vi "Untitled 1.vi"() -> ()   [LabVIEW 2016]
uses:
  BuildItem.ctl
  <vilib>/addons/_JKI.lib/Serialization/JSON/JKI JSON Serialization.lvlib
panel:
  in  "EnableAll":bool
  in  "DisableAll":bool
  in  "Cluster":cluster{"Enable":bool, "BuildItem":T1}={"Enable"=TRUE, "BuildItem"={"Project"=path "", "BuildSpecification"=path "", "Destination"=path ""}}
  in  "OK Button":bool
  in  "Array":cluster{"Enable":bool, "BuildItem":T1}[](array[cluster])
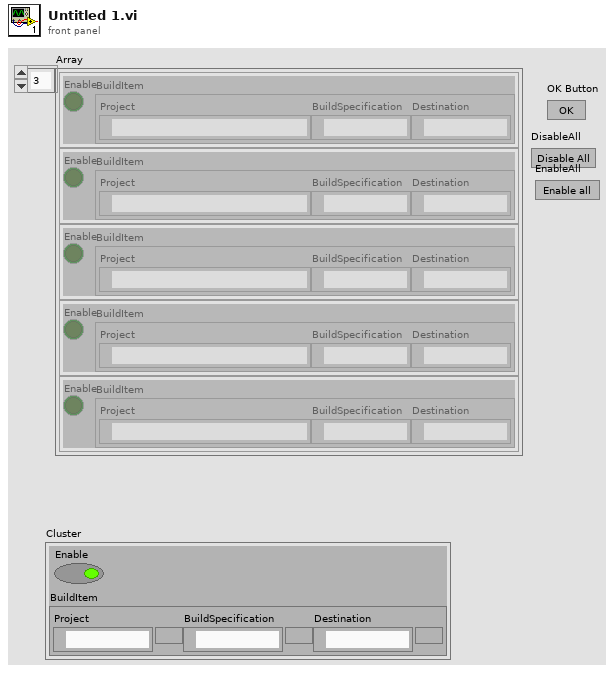
[diagram p1: front panel]
types:
  T1 = typedef "BuildItem.ctl" = cluster{"Project":path, "BuildSpecification":path, "Destination":path}
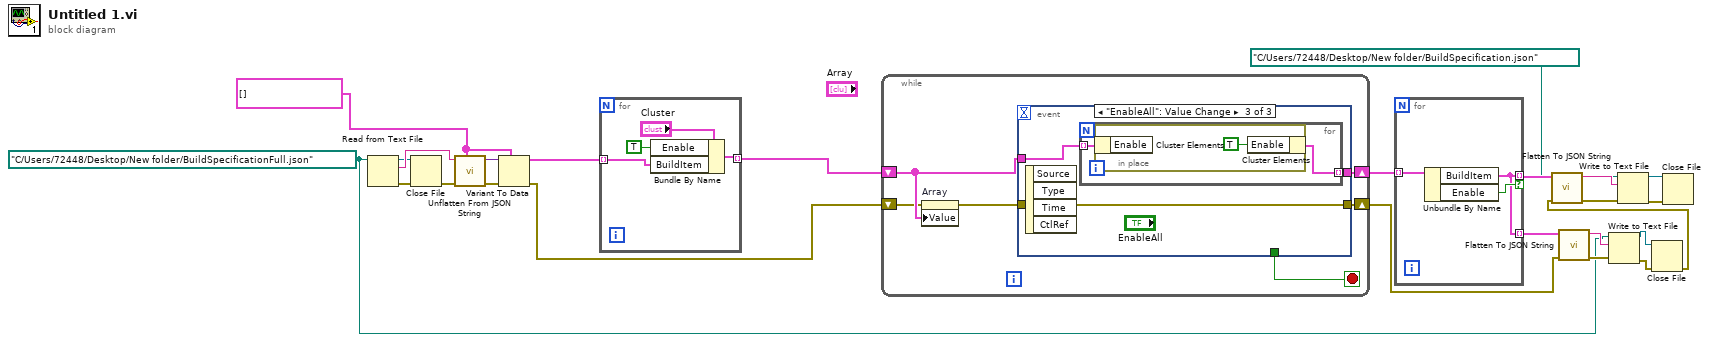
[diagram p0: block diagram]
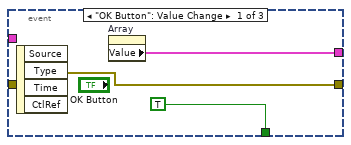
[diagram p2: hidden frame]
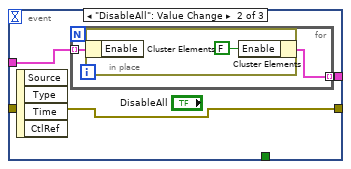
[diagram p3: hidden frame]
diagram:
  w18 = T1[] []
  w4 = path "C:/Users/72448/Desktop/New folder/BuildSpecificationFull.json" ("file (use dialog)")
  n1 = Read from Text File(file (use dialog)=w4) -> (refnum out=w20:refnum<file>, text=w23:string, error out=w21:errorcluster)  [unwired: 3 in, 1 out]
  n2 = Close File(refnum=w20, error in=w21) -> (error out=w22:errorcluster)  [unwired: 1 out]
  n3 = call <vilib>:"Unflatten From JSON String.vi"("Type and Defaults"=w18, "error in (no error)"=w22, "JSON String"=w23) -> ("error out"=w25:errorcluster, "Variant"=w24:variant)  [unwired: 7 in]
  n4 = Variant To Data(error in=w25, type=w18, Variant=w24) -> (data=w19:T1[], error out=w7:errorcluster)
  n5 = for {
    tunnel: w19 -> [w28] mode=indexing
    tunnel: [w26] -> w10 mode=indexing
    n6 = Bundle By Name(cluster="Cluster", "Enable"=TRUE, "BuildItem"=w28) -> (w26:cluster{"Enable":bool, "BuildItem":T1})
  }
  n7 = while {
    shift-right: [w35] -> w17
    shift-left: w10 -> [w33]
    shift-right: [w31] -> w8
    shift-left: w7 -> [w30]
    stop <- w34 stop-if-true
    n8 = property on="Array" class="Arr (strict)"(error in=w30, "Value"=w33) -> (error out=w32:errorcluster)  [unwired: 1 in, 1 out]
    n9 = event shown="[2] \"EnableAll\": Value Change" {
      selector: _ -> [_ _ _]
      dyn-events: _ -> [_ _ _]
      timeout: _ -> [_ _ _]
      tunnel: [w38 w40 w46] -> w35
      tunnel: w33 -> [_ w41 w47]
      tunnel: [TRUE _ _] -> w34
      tunnel: w32 -> [w36 w39 w45]
      tunnel: [w36 w39 w45] -> w31
      event "OK Button": Value Change {
        n10 = event-data() -> ()  [unwired: 1 in, 4 out]
        n11 = property on="Array" class="Arr (strict)"() -> ("Value"=w38:cluster{"Enable":bool, "BuildItem":T1}[])  [unwired: 2 in, 2 out]
      }
      event "DisableAll": Value Change {
        n12 = event-data() -> ()  [unwired: 1 in, 4 out]
        n13 = for {
          tunnel: w41 -> [w43] mode=indexing
          tunnel: [w42] -> w40 mode=indexing
          n14 = in-place {
            n15 = in-place-cluster #1(w43) -> ()  [unwired: 1 out]
            n16 = in-place-cluster #1("Enable"=FALSE) -> (w42:cluster{"Enable":bool, "BuildItem":T1})
          }
        }
      }
      event "EnableAll": Value Change {
        n17 = event-data() -> ()  [unwired: 1 in, 4 out]
        n18 = for {
          tunnel: w47 -> [w49] mode=indexing
          tunnel: [w48] -> w46 mode=indexing
          n19 = in-place {
            n20 = in-place-cluster #2(w49) -> ()  [unwired: 1 out]
            n21 = in-place-cluster #2("Enable"=TRUE) -> (w48:cluster{"Enable":bool, "BuildItem":T1})
          }
        }
      }
    }
  }
  n22 = for {
    tunnel: w17 -> [w53] mode=indexing
    tunnel: [w51] -> w16 mode=indexing if=w52
    tunnel: [w51] -> w9 mode=indexing
    n23 = Unbundle By Name(w53) -> ("BuildItem"=w51:T1, "Enable"=w52:bool)
  }
  n24 = call <vilib>:"Flatten To JSON String.vi"("error in (no error)"=w8, "Variant"=w9) -> ("error out"=w6:errorcluster, "JSON String"=w5:string)  [unwired: 8 in]
  n25 = Write to Text File(file (use dialog)=w4, text=w5, error in=w6) -> (refnum out=w3:refnum<file>, error out=w2:errorcluster)  [unwired: 1 in, 1 out]
  n26 = Close File(refnum=w3, error in=w2) -> (error out=w1:errorcluster)  [unwired: 1 out]
  n27 = call <vilib>:"Flatten To JSON String.vi"("error in (no error)"=w1, "Variant"=w16) -> ("error out"=w14:errorcluster, "JSON String"=w15:string)  [unwired: 8 in]
  n28 = Write to Text File(file (use dialog)=path "C:/Users/72448/Desktop/New folder/BuildSpecification.json", text=w15, error in=w14) -> (refnum out=w12:refnum<file>, error out=w13:errorcluster)  [unwired: 1 in, 1 out]
  n29 = Close File(refnum=w12, error in=w13) -> ()  [unwired: 2 out]
